vi "Decimate Profile.vi"(10 "Current Profile in":waveform(dbl)[](array[waveform]), 11 "Voltage Profile in":waveform(dbl)[](array[waveform])) -> (2 "Current Profile out":waveform(dbl)[](array[waveform]), 3 "Voltage Profile out":waveform(dbl)[](array[waveform]))   [LabVIEW 2023, in "EIS.lvclass"]
uses:
  EIS.lvclass
  EIS.lvclass/EIS.ctl
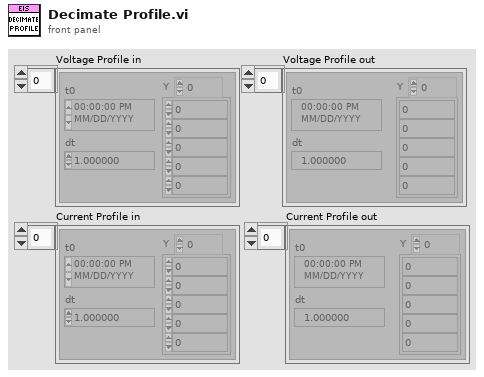
[diagram p1: front panel]
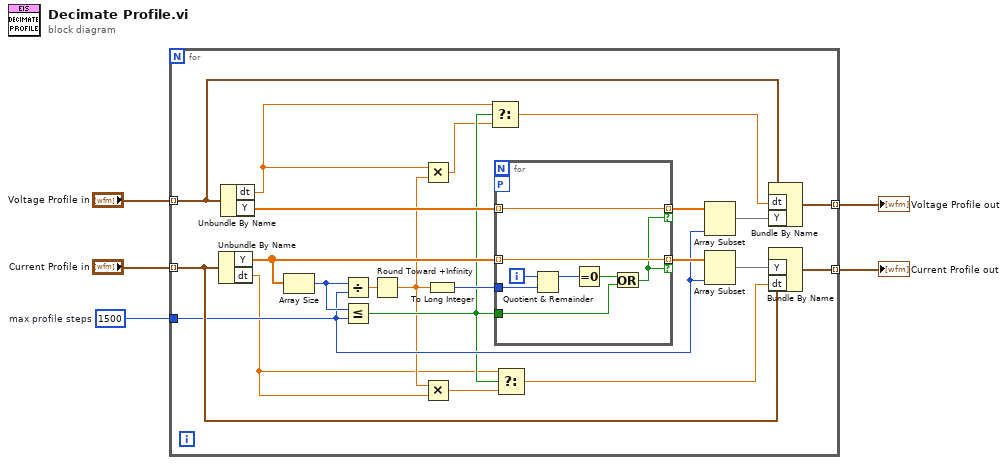
[diagram p0: block diagram]
diagram:
  w1 = 1500  # max profile steps
  n1 = for {
    tunnel: "Voltage Profile in" -> [w27] mode=indexing
    tunnel: "Current Profile in" -> [w25] mode=indexing
    tunnel: [w26] -> w3 mode=indexing
    tunnel: [w24] -> w2 mode=indexing
    tunnel: w1 -> [w14]
    n2 = Unbundle By Name(w25) -> ("Y"=w20:dbl[], "dt"=w7:dbl)
    n3 = Unbundle By Name(w27) -> ("dt"=w10:dbl, "Y"=w21:dbl[])
    n4 = Array Size(array=w20) -> (size(s)=w19:i32)
    n5 = Divide(x=w19, y=w14) -> (x/y=w22:dbl)
    n6 = Less Or Equal?(x=w19, y=w14) -> (x <= y?=w13:bool)
    n7 = Round Toward +Infinity(x=w22) -> (ceil(x): smallest int >= x=w8:dbl)
    n8 = Multiply(x=w10, y=w8) -> (x*y=w9:dbl)
    n9 = Multiply(x=w8, y=w7) -> (x*y=w6:dbl)
    n10 = To Long Integer(number=w8) -> (32bit integer=w23:i32)
    n11 = Select(t=w10, s=w13, f=w9) -> (s? t:f=w11:dbl)
    n12 = for {
      tunnel: w20 -> [w30] mode=indexing
      workers-P: _ -> [_]
      tunnel: w23 -> [w34]
      tunnel: w13 -> [w31]
      tunnel: w21 -> [w29] mode=indexing
      tunnel: [w30] -> w17 mode=indexing if=w28
      tunnel: [w29] -> w16 mode=indexing if=w28
      i -> [w35]
      n13 = Quotient & Remainder(x=w35, y=w34) -> (x-y*floor(x/y)=w33:i32)  [unwired: 1 out]
      n14 = Equal To 0?(x=w33) -> (x = 0?=w32:bool)
      n15 = Or(x=w32, y=w31) -> (x .or. y?=w28:bool)
    }
    n16 = Select(t=w7, s=w13, f=w6) -> (s? t:f=w18:dbl)
    n17 = Array Subset(array=w16, length=w14) -> (w15:dbl[])  [unwired: 1 in]
    n18 = Array Subset(array=w17, length=w14) -> (w12:dbl[])  [unwired: 1 in]
    n19 = Bundle By Name(cluster=w27, "dt"=w11, "Y"=w15) -> (w26:waveform(dbl))
    n20 = Bundle By Name(cluster=w25, "Y"=w12, "dt"=w18) -> (w24:waveform(dbl))
  }
  "Voltage Profile out" <- w3
  "Current Profile out" <- w2
